vi "Master Setup Update to RT.vi"(4 "error in (no error)":errorcluster, 5 "Pattern Label":T1 items=["Channel Setup (0)", "PID Setup (1)", "Filter Setup (2)", "~Reserved Old CAN Msgs (3)", "~Reserved Old CAN1 (4)", "~Reserved Old CAN2 (5)", "Digital Inputs Setup (6)", "Digital Outputs Setup (7)", "Logging 1 Setup (8)", "Logging 2 Setup (9)", "Logging 3 Setup (10)", "Setpoint Setup (11)", "Test Series Setup (12)", "Graph Setup (13)", "System Configure (14)", "Header (15)", "Profile Manager (16)", "Post-Mortem Logging (17)", "High-Speed Data (18)", "Statistic Channel Setup (19)", "Ramp Channel Setup (20)", "ETAS INCA Channel Setup (21)", "ETC ECCS Transducer Setup (22)", "ETC ECCS Test Setup (23)", "AVL AK Smoke Meter Setup (24)", "Triggers Setup (25)", "Alarm Limits Setup (26)", "YKWT1 Measurement (27)", "YKWT1 Instrument (28)", "Auto File Settings (29)", "Playback File Setting (30)", "UUT Constants (31)", "UPS Setup (32)", "Differential Channel Setup (33)", "Integral Channel Setup (34)", "Signal Channel Setup (35)", "Calibration Setup (36)", "BNC Setup (37)", "ASAP3 Setup (38)", "Chassis Force Calculations (39)", "Chassis Teststand Losses (40)", "Chassis Vehicle Losses (41)", "Formula Channels (42)", "ASAP3 Map Coords Setup (43)", "Digital Controls Setup (44)", "Push Buttons Setup (45)", "Sliders Setup (46)", "~Reserved~ (47)", "Email Setup (48)", "Timer Setup (49)", "Unit Conversion Setup (50)", "Visible Channels (51)", "Main Display Setup (52)", "Message Display Setup (53)", "Input Display Setup (54)", "Unico Parameter Downloads (55)", "Flow Meter Setup (56)", "Channel Zero Offset (57)", "YKWT2 Measurement (58)", "YKWT2 Instrument (59)", "~Reserved Old CAN3 (60)", "CAS Setup (61)", "Accumulation Channel Setup (62)", "Valvetrain Dynamics Setup (63)", "CCP Setup (64)", "System Log Setup (65)", "Throttle Controller (66)", "RE Shifter (67)", "Main Display (68)", "~Reserved~ (69)", "FlexRay (70)", "YKWT3 Measurement (71)", "YKWT3 Instrument (72)", "CAN XNET API (73)"], 7 "Setup String":string) -> (0 "error out":errorcluster)   [LabVIEW 2017]
uses:
  Master Setup Pattern Enum.ctl
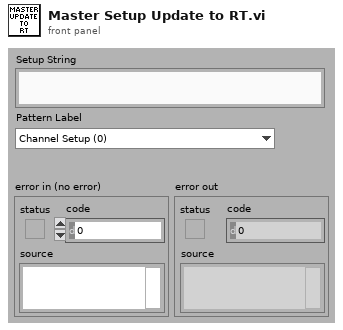
[diagram p1: front panel]
types:
  T1 = typedef "Master Setup Pattern Enum.ctl" = i32
  T2 = enum16{"1. Write to PC Network Shared Variable", "2. Command Real-Time to Update", "3. Wait Real-Time Update to Reset", "4. Check RT Network Shared Variable"}
  T3 = typedef "PC_INI_Data__TypeDef.ctl" = cluster{"REPS Version":T4, "System Configuration":T5, "OPC PLC Write":string, "OPC PLC Read":string, "Modbus Info":string, "INCA Configuration":cluster{"IP":string, "Port":i32, "Protocol Version":i32}, "ECCS Setup":cluster{"Enable":bool, "IP":string, "TCP Port":u16, "UDP Port":u16, "Engine ODBC Name":string, "Fuel ODBC Name":string}, "Encoder Configuration":cluster{"Encoder1PPR":i32, "Encoder1Interval1":i32, "Encoder1Interval2":i32, "Roll Diameter(Feet)":i32, "Encoder2PPR":i32, "Encoder3PPR":i32, "Encoder4PPR":i32, "Encoder5PPR":i32, "Encoder2Interval1":i32, "Encoder2Interval2":i32, "Encoder3Interval1":i32, "Encoder3Interval2":i32}, "Pickup1 Configuration":cluster{"PickupPPR":i32, "PickupInterval1":i32, "PickupInterval2":i32}, "Pickup2 Configuration":cluster{"PickupPPR":i32, "PickupInterval1":i32, "PickupInterval2":i32}, "Pickup3 Configuration":cluster{"PickupPPR":i32, "PickupInterval1":i32, "PickupInterval2":i32}, "Shifter Configuration":cluster{"RE Shifter Enable":bool, "Shifter IP Address":string, "Shifter Port":u16}, "Misc Configuration":T6, "Logging Configuration":cluster{"Number of Log Channels":dbl, "Max Log  File Size":dbl}}
  T4 = typedef "REPS Version.ctl" = cluster{"Version":string}
  T5 = typedef "System Configuration.ctl" = cluster{"Cell":string, "DualMotorSet":bool, "Hardware Setup Array":bool[], "Host IP":string, "Remote IP 1":string, "Remote IP 2":string, "Remote IP 3":string, "Remote Enable 1":bool, "Remote Enable 2":bool, "Remote Enable 3":bool, "Company Name":string, "Company Info":string, "Number Of Modbus":i32, "Setup Files Path":path, "Master File Path":path, "Master Setup Titles":string[], "Encoder1PPR":i32, "Encoder1Interval1":i32, "Encoder1Interval2":i32, "Display File Error Status?":bool[], "Update to RT Delay":u32, "Formula Rate (Hz)":u32, "Custom Screen (Left) Path":path, "Custom Screen (Right) Path":path}
  T6 = typedef "Misc Configuration.ctl" = cluster{"Show PM Logging Indicator":bool}
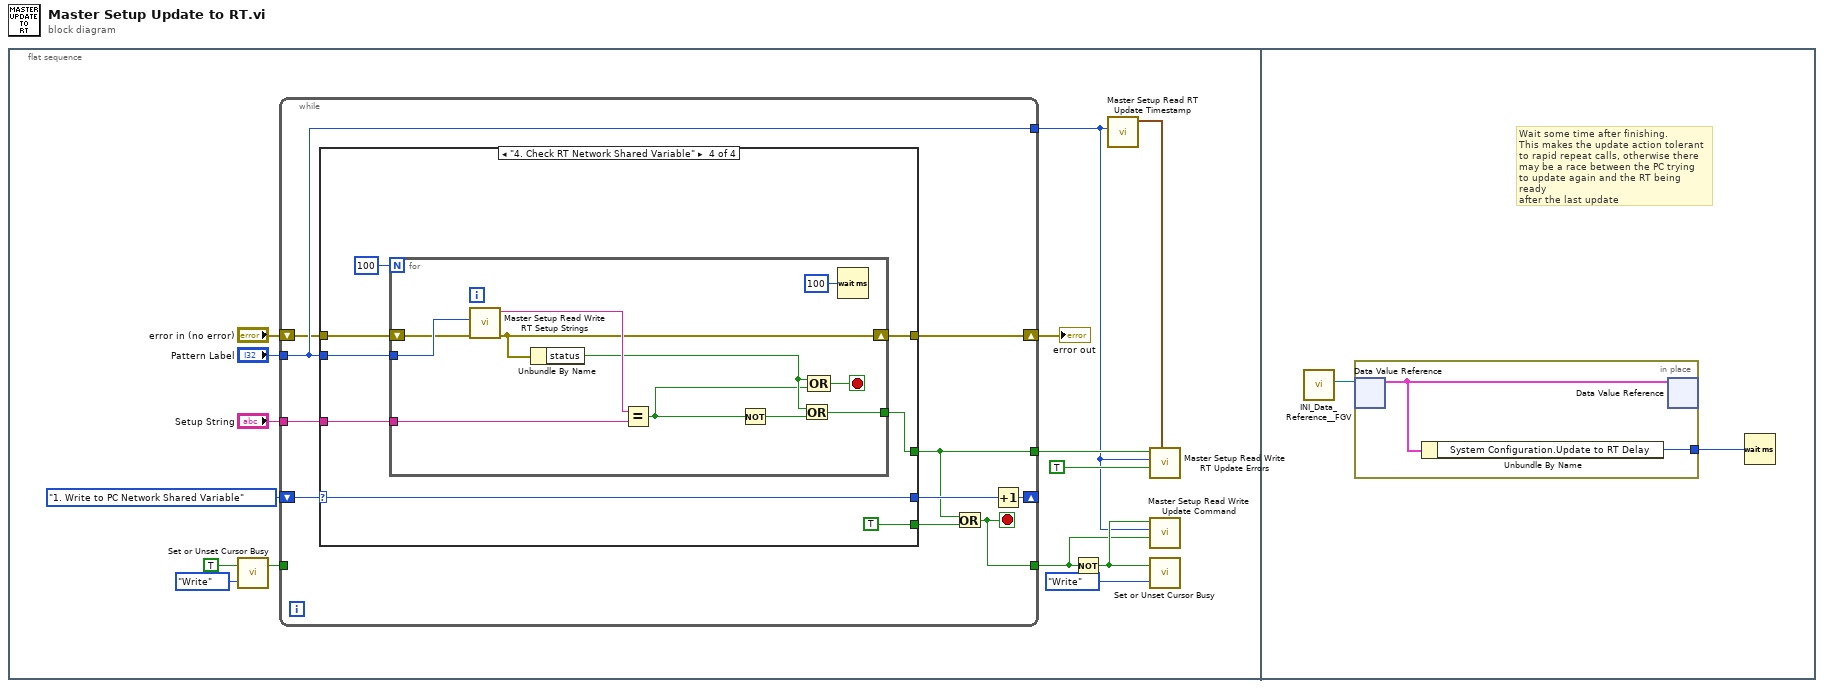
[diagram p0: block diagram]
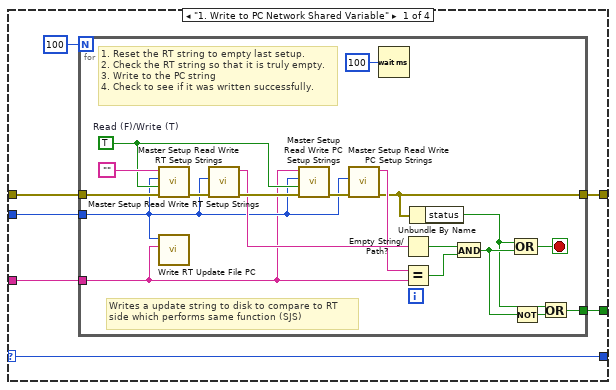
[diagram p2: hidden frame]
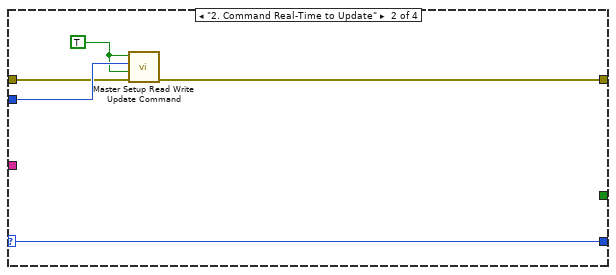
[diagram p3: hidden frame]
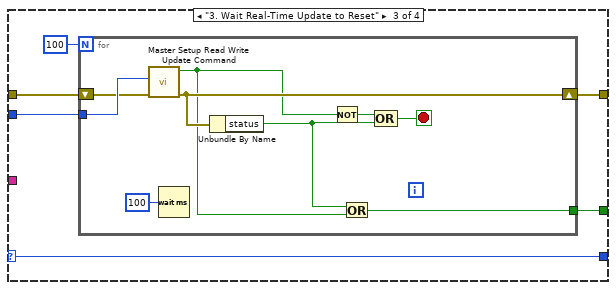
[diagram p4: hidden frame]
diagram:
  n1 = flat-sequence {
    frame #0 {
      n2 = call "Set or Unset Cursor Busy.vi"("Function (read)"=enum16{"Create", "Write", "Read", "Destroy"}."Write", "Cursor Busy (in)"=TRUE) -> ("Cursor Busy (out)"=w8:bool)  [unwired: 1 out]
      n3 = while {
        tunnel: "Setup String" -> [w25]
        tunnel: [w20] -> w13
        shift-right: [w22] -> _
        shift-left: T2."1. Write to PC Network Shared Variable" -> [w23]
        tunnel: w8 -> [_]
        tunnel: [w19] -> w4
        tunnel: "Pattern Label" -> [w18]
        tunnel: [w18] -> w3
        shift-right: [w17] -> w1
        shift-left: "error in (no error)" -> [w16]
        stop <- w19 stop-if-true
        n4 = case shown="\"4. Check RT Network Shared Variable\"" w23 {
          selector: w23 -> [w31 w56 w61 w78]
          tunnel: w25 -> [w32 _ _ w79]
          tunnel: [w26 _ w62 w72] -> w20
          tunnel: [w31 w56 w61 w78] -> w24
          tunnel: [_ _ _ TRUE] -> w21
          tunnel: w18 -> [w30 w55 w60 w76]
          tunnel: [w29 w52 w58 w74] -> w17
          tunnel: w16 -> [w28 w53 w59 w75]
          frame "1. Write to PC Network Shared Variable" {
            n5 = for {
              N: 100 -> [_]
              tunnel: w32 -> [w33]
              tunnel: w30 -> [w34]
              tunnel: [w40] -> w29
              tunnel: w28 -> [w41]
              tunnel: [w36] -> w26
              stop <- w39 stop-if-true
              w44 = TRUE  # Read (F)/Write (T)
              # "Writes a update string to disk to compare to RT\nside which performs same function (SJS)"
              # "1. Reset the RT string to empty last setup.\n2. Check the RT string so that it is truly empty.\n3. Write to the PC string\n4. Check to see if it was written successfully."
              n6 = call "Master Setup Read Write RT Setup Strings.vi"("error in (no error)"=w41, "Read (F)/Write (T)"=w44, "Pattern Label"=w34, "RT Setup String (in)"="") -> ("error out"=w47:errorcluster)  [unwired: 6 in, 1 out]
              n7 = call "Write RT Update File PC.vi"("Format String"=w33, "Pattern Label"=w34) -> ()  [unwired: 9 in, 1 out]
              n8 = call "Master Setup Read Write RT Setup Strings.vi"("error in (no error)"=w47, "Pattern Label"=w34) -> ("error out"=w46:errorcluster, "RT Setup String (out)"=w43:string)  [unwired: 8 in]
              n9 = call "Master Setup Read Write PC Setup Strings.vi"("error in (no error)"=w46, "Read (F)/Write (T)"=w44, "Pattern Label"=w34, "RT Setup String (in)"=w33) -> ("error out"=w45:errorcluster)  [unwired: 6 in, 1 out]
              n10 = call "Master Setup Read Write PC Setup Strings.vi"("error in (no error)"=w45, "Pattern Label"=w34) -> ("error out"=w40:errorcluster, "RT Setup String (out)"=w42:string)  [unwired: 8 in]
              n11 = Wait (ms)(milliseconds to wait=u32 100) -> ()  [unwired: 1 out]
              n12 = Empty String/Path?(string/path=w43) -> (empty?=w49:bool)
              n13 = Equal?(x=w42, y=w33) -> (x = y?=w51:bool)
              n14 = Unbundle By Name(w40) -> ("status"=w35:bool)
              n15 = And(x=w49, y=w51) -> (x .and. y?=w38:bool)
              n16 = Not(x=w38) -> (.not. x?=w37:bool)
              n17 = Compound Arithmetic op=OR(w35, w38) -> (w39:bool)
              n18 = Or(x=w35, y=w37) -> (x .or. y?=w36:bool)
            }
          }
          frame "2. Command Real-Time to Update" {
            w54 = TRUE ("Update Command - Playback Data")
            n19 = call "Master Setup Read Write Update Command.vi"("error in (no error)"=w53, "Read (F)/Write (T)"=w54, "Pattern Label"=w55, "Update Command (in)"=w54) -> ("error out"=w52:errorcluster)  [unwired: 6 in, 1 out]
          }
          frame "3. Wait Real-Time Update to Reset" {
            n20 = for {
              N: 100 -> [_]
              tunnel: [w64] -> w62
              tunnel: w60 -> [w69]
              shift-right: [w67] -> w58
              shift-left: w59 -> [w68]
              stop <- w66 stop-if-true
              n21 = call "Master Setup Read Write Update Command.vi"("error in (no error)"=w68, "Pattern Label"=w69) -> ("error out"=w67:errorcluster, "Update Command (out)"=w65:bool)  [unwired: 8 in]
              n22 = Wait (ms)(milliseconds to wait=u32 100) -> ()  [unwired: 1 out]
              n23 = Unbundle By Name(w67) -> ("status"=w63:bool)
              n24 = Not(x=w65) -> (.not. x?=w70:bool)
              n25 = Or(x=w63, y=w65) -> (x .or. y?=w64:bool)
              n26 = Compound Arithmetic op=OR(w70, w63) -> (w66:bool)
            }
          }
          frame "4. Check RT Network Shared Variable" {
            n27 = for {
              N: 100 -> [_]
              tunnel: w79 -> [w89]
              tunnel: w76 -> [w88]
              shift-right: [w85] -> w74
              shift-left: w75 -> [w86]
              tunnel: [w80] -> w72
              stop <- w84 stop-if-true
              n28 = call "Master Setup Read Write RT Setup Strings.vi"("error in (no error)"=w86, "Pattern Label"=w88) -> ("error out"=w85:errorcluster, "RT Setup String (out)"=w87:string)  [unwired: 8 in]
              n29 = Unbundle By Name(w85) -> ("status"=w83:bool)
              n30 = Equal?(x=w87, y=w89) -> (x = y?=w82:bool)
              n31 = Not(x=w82) -> (.not. x?=w81:bool)
              n32 = Or(x=w83, y=w81) -> (x .or. y?=w80:bool)
              n33 = Compound Arithmetic op=OR(w83, w82) -> (w84:bool)
              n34 = Wait (ms)(milliseconds to wait=u32 100) -> ()  [unwired: 1 out]
            }
          }
        }
        n35 = Or(x=w20, y=w21) -> (x .or. y?=w19:bool)
        n36 = Increment(x=w24) -> (x+1=w22:T2)
      }
      "error out" <- w1
      n37 = Not(x=w4) -> (.not. x?=w5:bool)
      n38 = call "Master Setup Read RT Update Timestamp.vi"("Pattern Label"=w3) -> ("RT Setup String (out)"=w6:timestamp)  [unwired: 9 in, 1 out]
      n39 = call "Master Setup Read Write RT Update Errors.vi"("RT Update Timestamp"=w6, "Read (F) Write (T)"=TRUE, "Pattern Label"=w3, "Error Status"=w13) -> ()  [unwired: 5 in, 3 out]
      n40 = call "Master Setup Read Write Update Command.vi"("Read (F)/Write (T)"=w4, "Pattern Label"=w3, "Update Command (in)"=w5) -> ()  [unwired: 7 in, 2 out]
      n41 = call "Set or Unset Cursor Busy.vi"("Function (read)"=enum16{"Create", "Write", "Read", "Destroy"}."Write", "Cursor Busy (in)"=w5) -> ()  [unwired: 2 out]
    }
    frame #1 {
      # "Wait some time after finishing.\nThis makes the update action tolerant\nto rapid repeat calls, otherwise there\nmay be a race between the PC trying\nto update again and the RT being ready\nafter the last update"
      n42 = call "INI_Data_Reference__FGV.vi"() -> (".ini Data Value Reference (out)"=w92:refnum<data-value>)  [unwired: 11 in]
      n43 = in-place {
        in-place-border: [w93] -> w91
        n44 = in-place-dvr #1(w92) -> (w94:T3)  [unwired: 1 out]
        n45 = Unbundle By Name(w94) -> ("System Configuration.Update to RT Delay"=w93:u32)
        n46 = in-place-dvr #1(w94) -> ()  [unwired: 2 out]
      }
      n47 = Wait (ms)(milliseconds to wait=w91) -> ()  [unwired: 1 out]
    }
  }
